vi "Algorithm.vi"(7 "Name(\"\" to use uuid)":string="CSM-Module") -> ()   [LabVIEW 2017, in "Algorithm.lvlib"]
uses:
  Algorithm.lvlib
  b0911fd4-62c2-45de-bc24-cb3c3c9cfef9.vi
  650347b4-7247-415a-b210-2ec4f3372018.vi
  d54ebfec-1730-4eff-a376-8c753df15871.vi
  08833c2f-3e6e-47d2-ae0f-0995abdd27de.vi
  d6c98f61-f9a9-4815-af94-1514c1bd458f.vi
  11c34204-1abb-4db0-9e93-68fba18ec886.vi
  fe892ae6-a90b-4c60-af4d-0c04454fd8c0.vi
  6b00cd4a-b76d-4b12-b38d-c43ef07dbd87.vi
  <userlib>/_NEVSTOP/Communicable State Machine(CSM)/AdvanceAPI/CSM - Revert Arguments-Safe String.vi
  <userlib>/_NEVSTOP/Communicable State Machine(CSM)/_Shared/Trim Single-line Text.vi
  <userlib>/_NEVSTOP/Communicable State Machine(CSM)/AdvanceAPI/CSM - Make String Arguments Safe.vi
  <userlib>/_NEVSTOP/Communicable State Machine(CSM)/AdvanceAPI/CSM - Break Down Multiple States String.vi
  <userlib>/_NEVSTOP/Communicable State Machine(CSM)/AdvanceAPI/CSM - Compact Multiple States.vi
  <userlib>/_NEVSTOP/Communicable State Machine(CSM)/AdvanceAPI/CSM - Keywords.vi
  <userlib>/_NEVSTOP/Communicable State Machine(CSM)/addons/API-String-Arugments-Support/_Support/Query Data as API String Arguments(variant).vi
  <userlib>/_NEVSTOP/Communicable State Machine(CSM)/addons/API-String-Arugments-Support/_Support/Convert API String Arguments to Data(variant).vi
  <userlib>/_NEVSTOP/Communicable State Machine(CSM)/addons/MassData-Parameter/_support/FGV-MassData(lvlibp).vi
  <vilib>/express/express analysis/Spectral/Block/exnSpectralBlock spectral measurements peak poly.vi
  <vilib>/express/express analysis/Spectral/Block/exnSpectralBlock spectral measurements peak array WFM.vi
  <vilib>/express/express analysis/Spectral/Block/exnSpectralBlock spectral measurements RMS poly.vi
  <vilib>/express/express analysis/Spectral/Block/exnSpectralBlock spectral measurements RMS array WFM.vi
  <vilib>/express/express analysis/Spectral/Block/exnSpectralBlock spectral measurements power poly.vi
  <vilib>/express/express analysis/Spectral/Block/exnSpectralBlock spectral measurements power array WFM.vi
  <vilib>/express/express analysis/Spectral/XNode/ExpressSpectralMeasurementsBlockNode.xnode
  <userlib>/_NEVSTOP/Communicable State Machine(CSM)/Communicable State Machine.lvlib
panel:
  out "Source":waveform(dbl)[](graph)
  out "Error Occurred":errorcluster
  out "State History":string
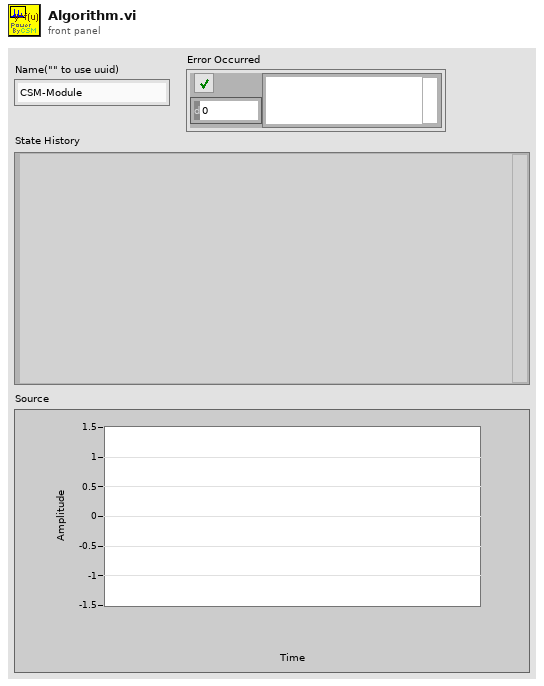
[diagram p1: front panel]
types:
  T1 = enum32{"Invalid", "Standard", "Closed", "Hidden", "Minimized", "Maximized"}
  T2 = enum32{"invalid app kind", "Development System", "Run Time System", "Student Edition", "Embedded LabVIEW", "Evaluation", "Custom"}
  T3 = cluster{"averaging mode":u16, "weighting mode":u16, "number of averages":u32}
  T4 = cluster{"dB On (F)":bool, "unwrap phase (F)":bool, "convert to degree (F)":bool}
  T5 = typedef "Communicable State Machine.lvlib/_CSM_Response Source Message.ctl" = cluster{"‘State":string, "’Arguments":string, "’Error":errorcluster}
  T6 = cluster{"Current VI Reference":refnum<vi>, "Close Panel on Exit?":bool}
  T7 = cluster{"Core":cluster{"Current VI Reference":refnum<vi>, "Close Panel on Exit?":bool}, "Your Boolean data":bool, "Your string data":string}
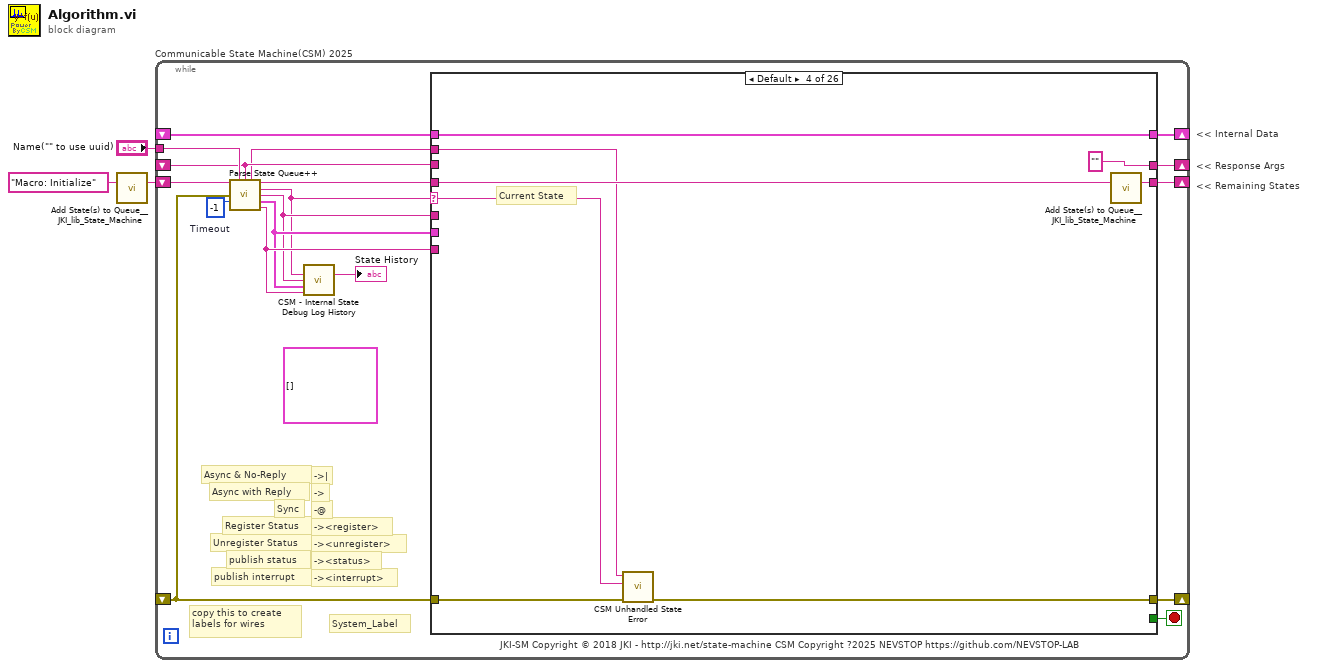
[diagram p0: block diagram]
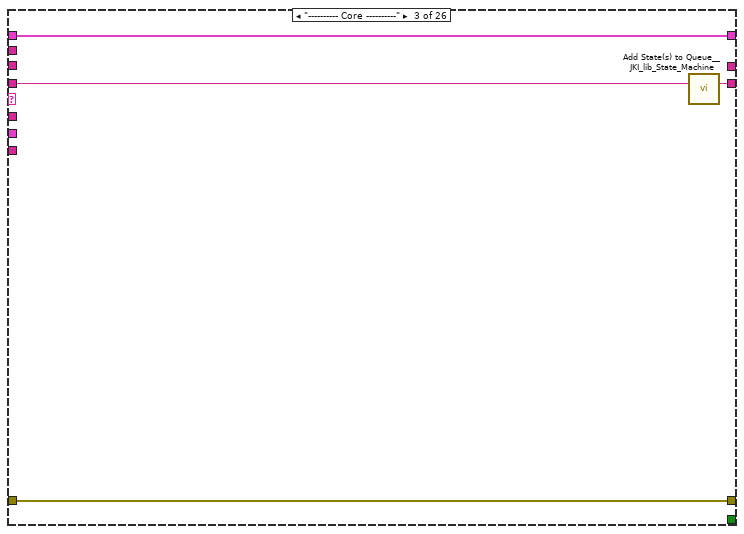
[diagram p4: hidden frame]
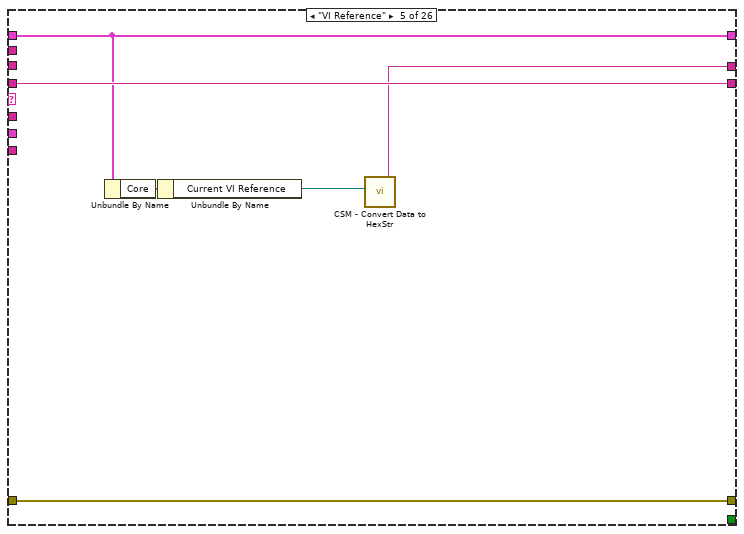
[diagram p5: hidden frame]
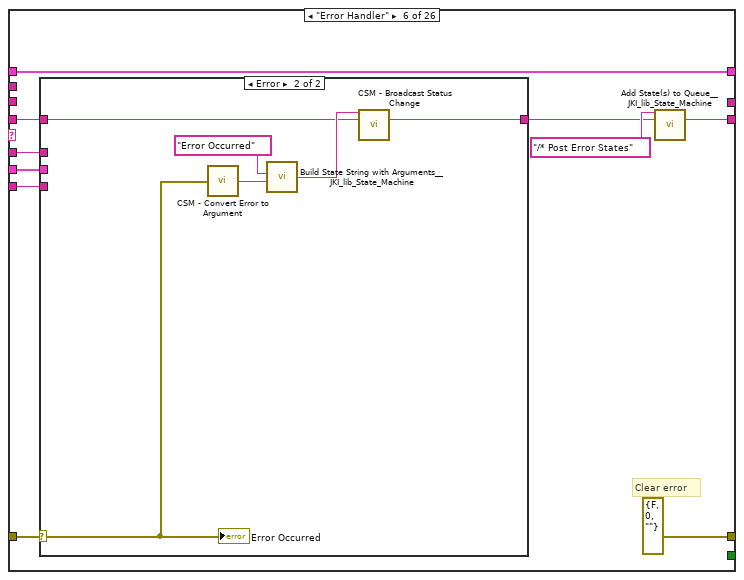
[diagram p6: hidden frame]
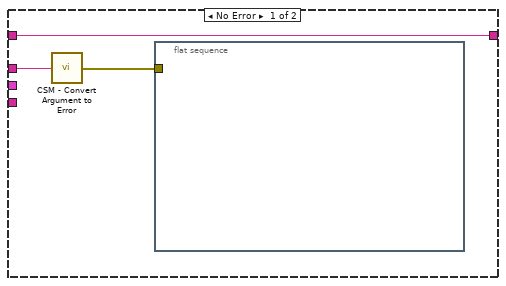
[diagram p7: hidden frame]
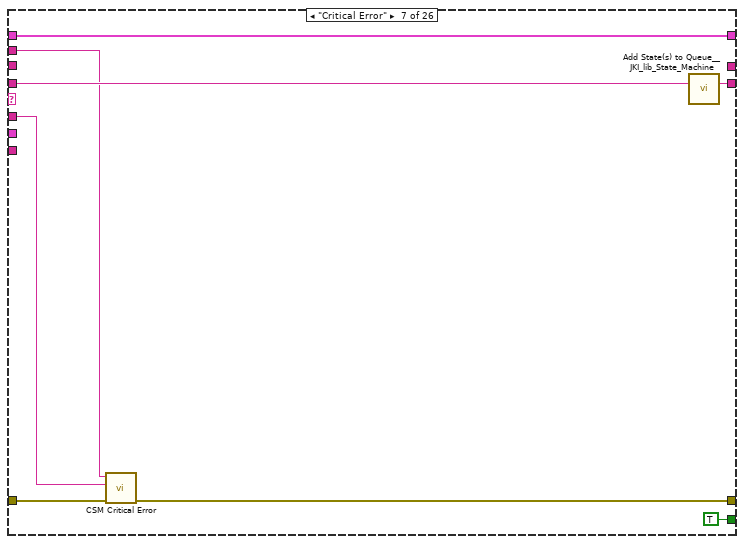
[diagram p8: hidden frame]
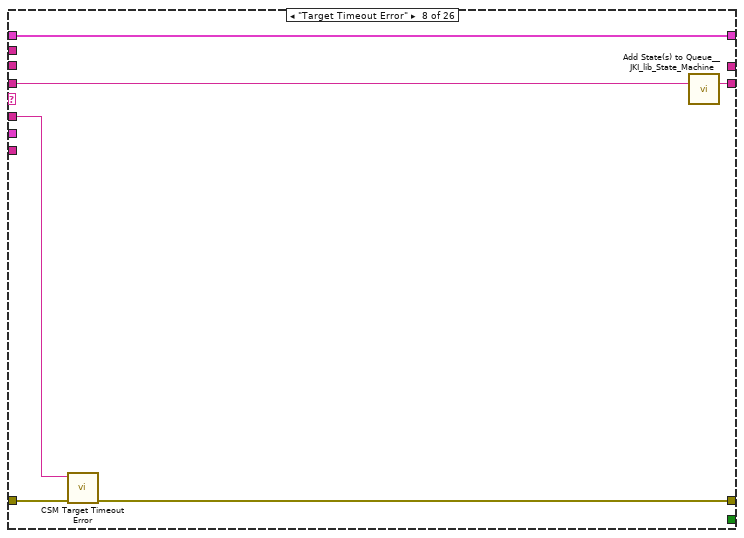
[diagram p9: hidden frame]
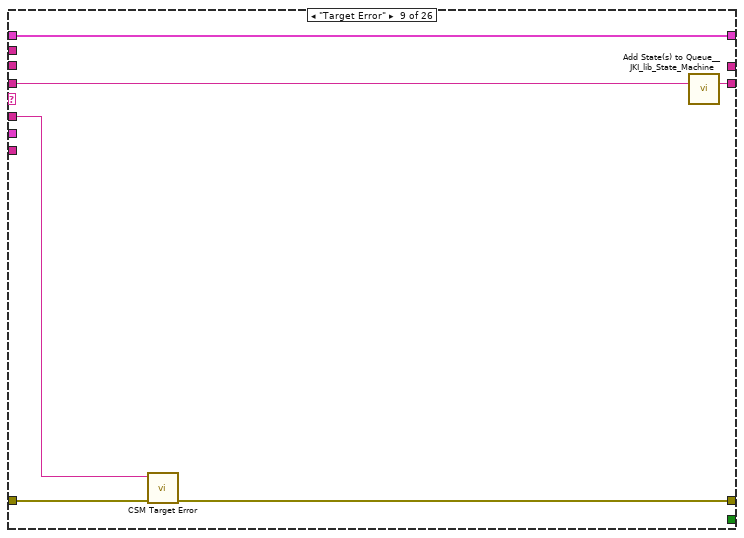
[diagram p10: hidden frame]
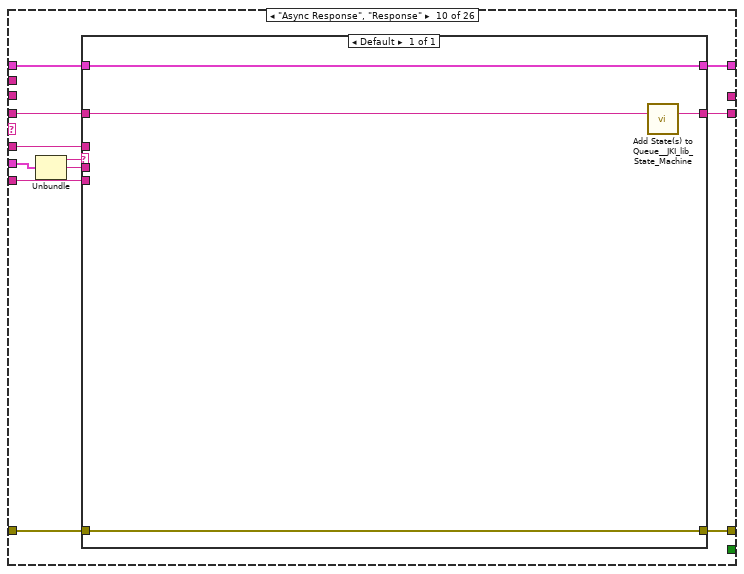
[diagram p11: hidden frame]
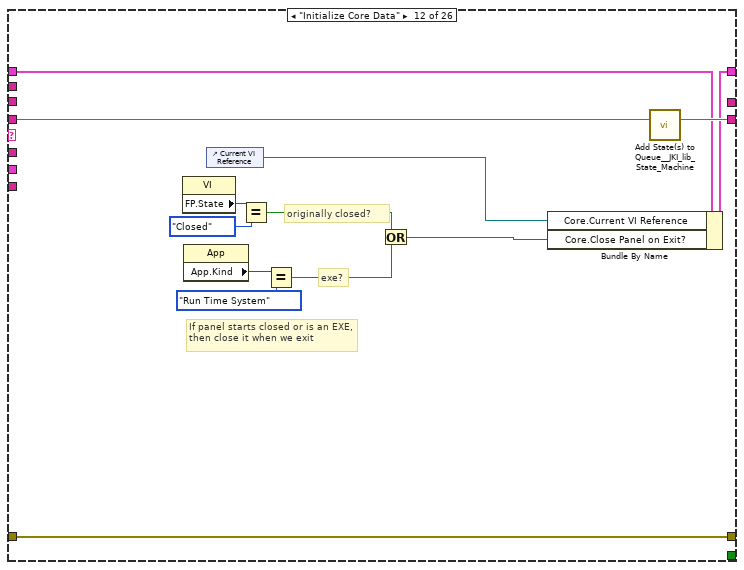
[diagram p13: hidden frame]
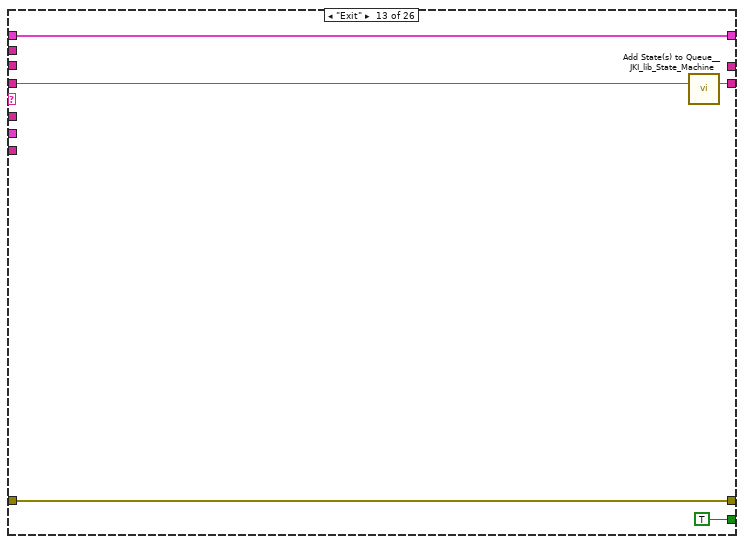
[diagram p14: hidden frame]
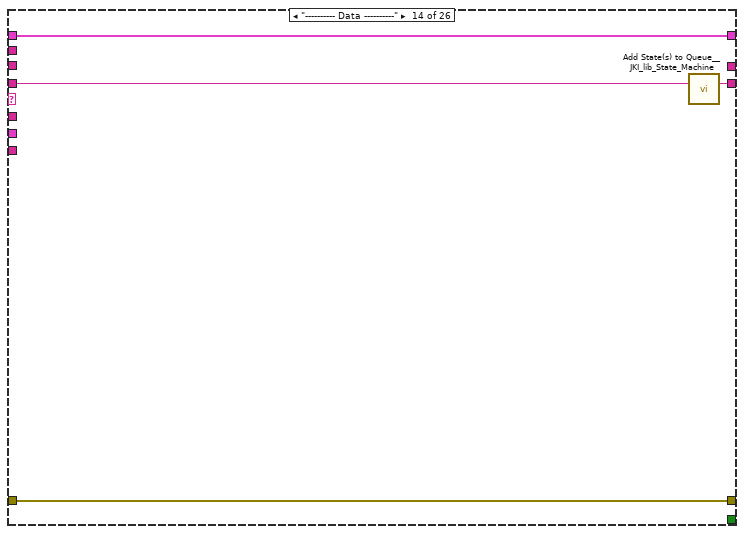
[diagram p15: hidden frame]
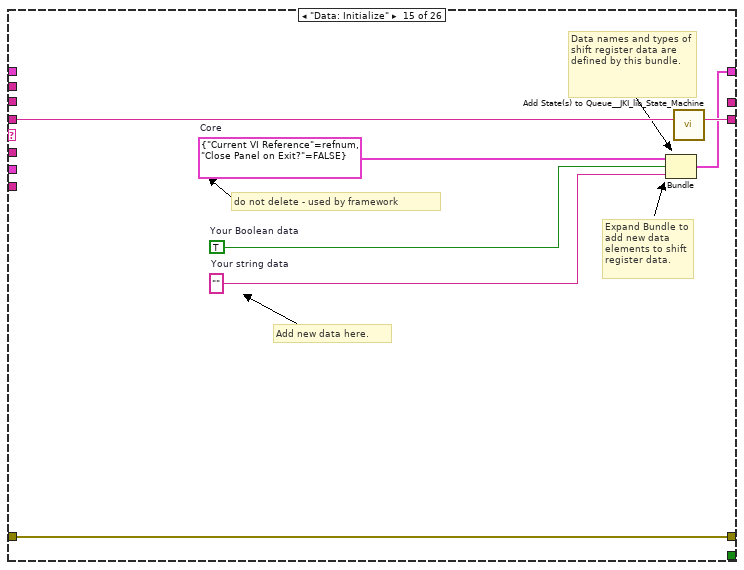
[diagram p16: hidden frame]
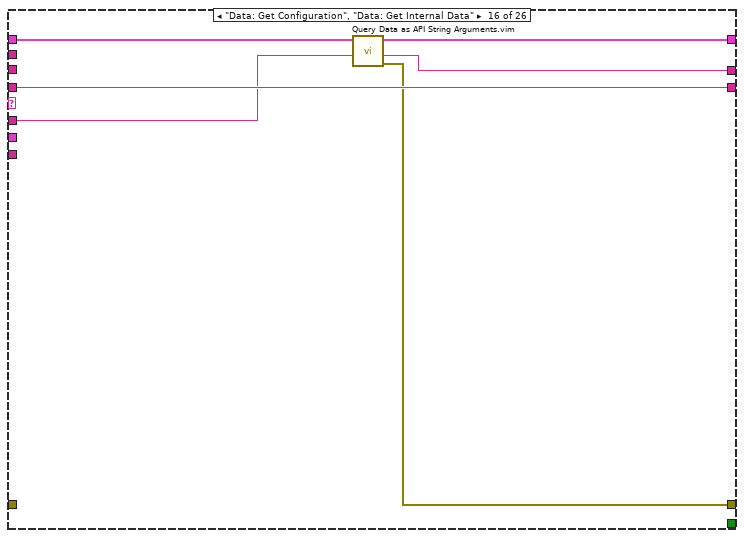
[diagram p17: hidden frame]
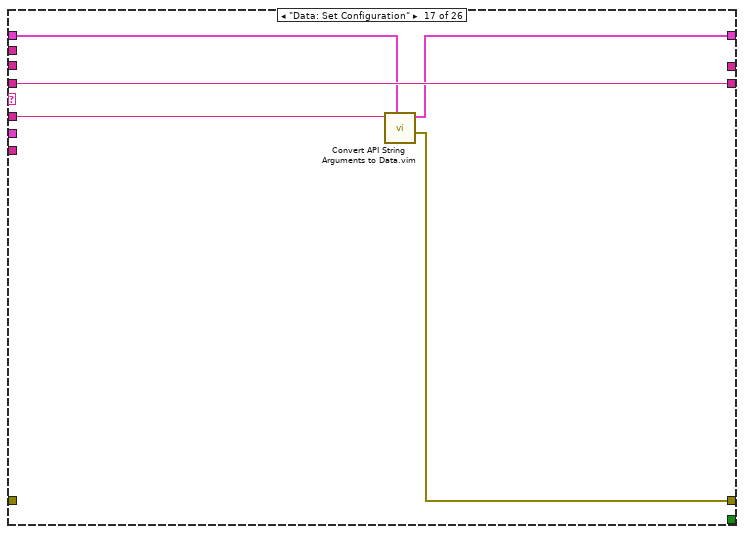
[diagram p18: hidden frame]
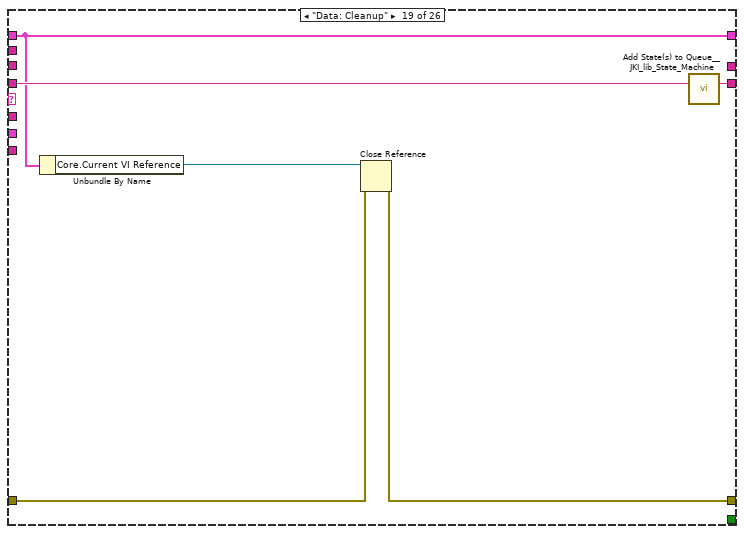
[diagram p20: hidden frame]
diagram:
  # "<< Internal Data"
  # "<< Response Args"
  # "<< Remaining States"
  n1 = call <vilib>:"Add State(s) to Queue__JKI_lib_State_Machine.vi"("State(s) in (\"\")"="Macro: Initialize") -> ("States Out"=w3:string)  [unwired: 14 in]
  n2 = while "Communicable State Machine(CSM) 2025" {
    shift-right: [w16] -> _
    shift-left: _ -> [w15]
    shift-right: [w19] -> _
    shift-left: _ -> [w5]
    shift-right: [w18] -> _
    shift-left: w3 -> [w20]
    tunnel: "Name(\"\" to use uuid)" -> [w12]
    shift-right: [w13] -> _
    shift-left: _ -> [w7]
    stop <- w17 stop-if-true
    (unwired) cluster{"f0":dbl, "df":dbl, "magnitude":dbl[]}[] [] ("FFT - (RMS)")
    w14 = -1  # Timeout
    # "copy this to create labels for wires"
    # "System_Label"
    # "-><interrupt>"
    # "-><status>"
    # "-><unregister>"
    # "-><register>"
    # "-@"
    # "->"
    # "->|"
    # "publish interrupt"
    # "publish status"
    # "Unregister Status"
    # "Register Status"
    # "Sync"
    # "Async with Reply"
    # "Async & No-Reply"
    # "JKI-SM Copyright © 2018 JKI - http://jki.net/state-machine CSM Copyright ?2025 NEVSTOP https://github.com/NEVSTOP-LAB"
    n3 = call <userlib>:"Parse State Queue++.vi"("State Queue"=w20, "Name (\"\" to Use UUID)"=w12, "Response Arguments"=w7, "Previous Error"=w5, "Dequeue (1 ms)"=w14) -> ("Name Used"=w6:string, "Remaining States"=w21:string, "Current State"=w8:string, "Arguments"=w9:string, "Additional Information"=w10:T5, "Source CSM"=w11:string)  [unwired: 5 in]
    n4 = call <userlib>:"CSM - Internal State Debug Log History.vi"("State"=w8, "Arguments (\"\")"=w9, ">> Response Source Message >>"=w10, "Source (\"\")"=w11) -> ("Debug Log"=→"State History":string)  [unwired: 11 in]
    n5 = case shown="Default" w8 {
      selector: w8 -> [_ _ _ w34 _ _ _ _ _ _ _ _ _ _ _ _ _ _ _ _ _ _ _ _ _ _]
      tunnel: w21 -> [w22 w26 w31 w38 w44 w49 w71 w77 w83 w88 w101 w115 w120 w124 w131 w137 w142 w144 w151 w155 w160 w165 w167 w178 w198 w218]
      tunnel: w9 -> [_ _ _ _ _ w48 w66 w74 w80 w87 _ _ _ _ _ w132 w141 _ _ _ _ _ _ w175 w195 w215]
      tunnel: w15 -> [w23 w25 w28 w36 w43 w54 w69 w75 w81 w89 w100 w108 w118 w121 _ w136 w140 w143 w146 w152 w157 w162 w166 w177 w197 w217]
      tunnel: [w24 w27 w29 w32 w45 errorcluster {"status"=FALSE, "code"=0, "source"=""} ("error out") w65 w73 w79 w92 w102 w112 w117 w122 w128 w133 w138 w145 w147 w153 w158 w163 w168 w171 w191 w211] -> w19
      tunnel: w5 -> [w24 w27 w29 w39 w45 w52 w72 w78 w84 w93 w102 w112 w117 w122 w128 _ _ w145 w148 w153 w158 w163 w168 _ _ _]
      tunnel: [w22 w26 w30 w37 w44 w50 w70 w76 w82 w90 w101 w114 w119 w123 w130 w137 w142 w144 w150 w154 w159 w164 w167 w178 w198 w218] -> w18
      tunnel: [_ _ _ _ _ _ TRUE _ _ _ _ _ TRUE _ _ _ _ _ _ _ _ _ _ _ _ _] -> w17
      tunnel: [w23 w25 w28 w36 w43 w54 w69 w75 w81 w91 w100 w113 w118 w121 w129 w135 w139 w143 w146 w152 w157 w162 w166 w177 w197 w217] -> w16
      tunnel: w11 -> [_ _ _ _ _ w47 _ _ _ w85 _ _ _ _ _ _ _ _ _ _ _ _ _ _ _ _]
      tunnel: w10 -> [_ _ _ _ _ w46 _ _ _ w86 _ _ _ _ _ _ _ _ _ _ _ _ _ _ _ _]
      tunnel: [_ _ _ "" w40 _ _ _ _ _ _ _ _ _ _ w134 _ _ _ _ _ _ _ w170 w190 w210] -> w13
      tunnel: w6 -> [_ _ _ w33 _ _ w67 _ _ _ _ _ _ _ _ _ _ _ _ _ _ _ _ _ _ _]
      tunnel: w7 -> [_ _ _ _ _ _ _ _ _ _ _ _ _ _ _ _ _ _ _ _ _ _ _ _ _ _]
      frame "", "Idle" {
      }
      frame "CSM Documentation" {
        # "CSM Documentation"
      }
      frame "---------- Core ----------" {
        n6 = call <vilib>:"Add State(s) to Queue__JKI_lib_State_Machine.vi"("State(s) in (\"\")"=w31) -> ("States Out"=w30:string)  [unwired: 14 in]
      }
      frame Default {
        # "Current State"
        n7 = call <userlib>:"CSM Unhandled State Error.vi"("error in (no error)"=w39, "Undefined State"=w34, "CSM Name"=w33) -> ("error out"=w32:errorcluster)  [unwired: 8 in]
        n8 = call <vilib>:"Add State(s) to Queue__JKI_lib_State_Machine.vi"("State(s) in (\"\")"=w38) -> ("States Out"=w37:string)  [unwired: 14 in]
      }
      frame "VI Reference" {
        n9 = Unbundle By Name(w43) -> ("Core"=w42:T6)
        n10 = Unbundle By Name(w42) -> ("Current VI Reference"=w41:refnum<vi>)
        n11 = call <userlib>:"CSM - Convert Data to HexStr.vi"("Variant"=w41) -> ("HEX String (0-9,A-F)"=w40:string)  [unwired: 8 in]
      }
      frame "Error Handler" {
        # "Clear error"
        n12 = case shown="Error" w52 {
          selector: w52 -> [_ w59]
          tunnel: [w58 w61] -> w51
          tunnel: w49 -> [w58 w60]
          tunnel: w48 -> [w57 _]
          tunnel: w47 -> [_ _]
          tunnel: w46 -> [_ _]
          frame No Error {
            n13 = call <userlib>:"CSM - Convert Argument to Error.vi"("Argument"=w57) -> ("Error"=w56:errorcluster)  [unwired: 4 in]
            n14 = flat-sequence {
              tunnel: w56 -> [_]
              frame #0 {
              }
            }
          }
          frame Error {
            n15 = call <userlib>:"CSM - Convert Error to Argument.vi"("Error"=w59) -> ("Argument"=w63:string)  [unwired: 4 in]
            n16 = call <vilib>:"Build State String with Arguments__JKI_lib_State_Machine.vi"("Arguments (\"\")"=w63, "State"="Error Occurred" ("Status with Arguments")) -> ("State with Arguments"=w62:string)  [unwired: 4 in]
            n17 = call <userlib>:"CSM - Broadcast Status Change.vi"("Status With Arguments"=w62, "State Queue"=w60) -> ("Remaining States"=w61:string)  [unwired: 13 in]
            "Error Occurred" <- w59
          }
        }
        n18 = call <vilib>:"Add State(s) to Queue__JKI_lib_State_Machine.vi"("State(s) in Front (\"\")"="/* Post Error States", "State(s) in (\"\")"=w51) -> ("States Out"=w50:string)  [unwired: 13 in]
      }
      frame "Critical Error" {
        n19 = call <userlib>:"CSM Critical Error.vi"("error in (no error)"=w72, "Arugments (As Reason)"=w66, "CSM Name"=w67) -> ("error out"=w65:errorcluster)  [unwired: 8 in]
        n20 = call <vilib>:"Add State(s) to Queue__JKI_lib_State_Machine.vi"("State(s) in (\"\")"=w71) -> ("States Out"=w70:string)  [unwired: 14 in]
      }
      frame "Target Timeout Error" {
        n21 = call <userlib>:"CSM Target Timeout Error.vi"("error in (no error)"=w78, "Arguments (As CSM Name)"=w74) -> ("error out"=w73:errorcluster)  [unwired: 9 in]
        n22 = call <vilib>:"Add State(s) to Queue__JKI_lib_State_Machine.vi"("State(s) in (\"\")"=w77) -> ("States Out"=w76:string)  [unwired: 14 in]
      }
      frame "Target Error" {
        n23 = call <userlib>:"CSM Target Error.vi"("error in (no error)"=w84, "Arguments (As CSM Name)"=w80) -> ("error out"=w79:errorcluster)  [unwired: 9 in]
        n24 = call <vilib>:"Add State(s) to Queue__JKI_lib_State_Machine.vi"("State(s) in (\"\")"=w83) -> ("States Out"=w82:string)  [unwired: 14 in]
      }
      frame "Async Response", "Response" {
        n25 = Unbundle(w86) -> ("‘State"=w95:string, "’Arguments"=w94:string)  [unwired: 1 out]
        n26 = case shown="Default" w95 {
          tunnel: [w96] -> w90
          tunnel: w88 -> [w97]
          tunnel: [w99] -> w91
          tunnel: w89 -> [w99]
          tunnel: [w98] -> w92
          tunnel: w93 -> [w98]
          tunnel: w85 -> [_]
          tunnel: w87 -> [_]
          tunnel: w94 -> [_]
          frame Default {
            n27 = call <vilib>:"Add State(s) to Queue__JKI_lib_State_Machine.vi"("State(s) in (\"\")"=w97) -> ("States Out"=w96:string)  [unwired: 14 in]
          }
        }
      }
      frame "Async Message Posted" {
      }
      frame "Initialize Core Data" {
        # "originally closed?"
        # "exe?"
        # "If panel starts closed or is an EXE, then close it when we exit"
        n28 = property class="VI"() -> ("FP.State"=w105:T1)  [unwired: 2 in, 2 out]
        n29 = property class="App"() -> ("App.Kind"=w111:T2)  [unwired: 2 in, 2 out]
        n30 = control-ref of="Current VI Reference"() -> (w106:refnum<vi>)
        n31 = Equal?(x=w105, y=T1."Closed" ("Front Panel Window:State")) -> (x = y?=w103:bool)
        n32 = Equal?(x=w111, y=T2."Run Time System" ("Application:Kind")) -> (x = y?=w109:bool)
        n33 = Or(x=w103, y=w109) -> (x .or. y?=w107:bool)
        n34 = Bundle By Name(cluster=w108, "Core.Current VI Reference"=w106, "Core.Close Panel on Exit?"=w107) -> (w113:T7)
        n35 = call <vilib>:"Add State(s) to Queue__JKI_lib_State_Machine.vi"("State(s) in (\"\")"=w115) -> ("States Out"=w114:string)  [unwired: 14 in]
      }
      frame "Exit" {
        n36 = call <vilib>:"Add State(s) to Queue__JKI_lib_State_Machine.vi"("State(s) in (\"\")"=w120) -> ("States Out"=w119:string)  [unwired: 14 in]
      }
      frame "---------- Data ----------" {
        n37 = call <vilib>:"Add State(s) to Queue__JKI_lib_State_Machine.vi"("State(s) in (\"\")"=w124) -> ("States Out"=w123:string)  [unwired: 14 in]
      }
      frame "Data: Initialize" {
        w125 = T6 {"Current VI Reference"=refnum, "Close Panel on Exit?"=FALSE}  # Core
        w127 = TRUE  # Your Boolean data
        w126 = ""  # Your string data
        # "do not delete - used by framework"
        # "Expand Bundle to add new data elements to shift register data."
        # "Add new data here."
        # "Data names and types of shift register data are defined by this bundle."
        n38 = Bundle("Core"=w125, "Your Boolean data"=w127, "Your string data"=w126) -> (w129:T7)  [unwired: 1 in]
        n39 = call <vilib>:"Add State(s) to Queue__JKI_lib_State_Machine.vi"("State(s) in (\"\")"=w131) -> ("States Out"=w130:string)  [unwired: 14 in]
      }
      frame "Data: Get Configuration", "Data: Get Internal Data" {
        n40 = call "Query Data as API String Arguments.vim"("Name"=w132, "Cluster Data"=w136) -> ("error"=w133:errorcluster, "API String"=w134:string, "Cluster Data (dup)"=w135:T7)  [unwired: 7 in]
      }
      frame "Data: Set Configuration" {
        n41 = call "Convert API String Arguments to Data.vim"("Reference Type"=w140, "API String"=w141) -> ("error out"=w138:errorcluster, "Data"=w139:T7)  [unwired: 6 in]
      }
      frame "Data: Update Indicators" {
      }
      frame "Data: Cleanup" {
        n42 = Unbundle By Name(w146) -> ("Core.Current VI Reference"=w149:refnum<vi>)
        n43 = Close Reference(reference=w149, error in (no error)=w148) -> (error out=w147:errorcluster)
        n44 = call <vilib>:"Add State(s) to Queue__JKI_lib_State_Machine.vi"("State(s) in (\"\")"=w151) -> ("States Out"=w150:string)  [unwired: 14 in]
      }
      frame "---------- Macro ----------" {
        n45 = call <vilib>:"Add State(s) to Queue__JKI_lib_State_Machine.vi"("State(s) in (\"\")"=w155) -> ("States Out"=w154:string)  [unwired: 14 in]
      }
      frame "Macro: Initialize" {
        n46 = call <vilib>:"Add State(s) to Queue__JKI_lib_State_Machine.vi"("State(s) in Front (\"\")"="Data: Initialize\nInitialize Core Data\nData: Update Indicators", "State(s) in (\"\")"=w160) -> ("States Out"=w159:string)  [unwired: 13 in]
      }
      frame "Macro: Exit" {
        n47 = call <vilib>:"Add State(s) to Queue__JKI_lib_State_Machine.vi"("State(s) in Front (\"\")"="Data: Cleanup\nExit", "State(s) in (\"\")"=w165) -> ("States Out"=w164:string)  [unwired: 13 in]
      }
      frame "---------- API ----------" {
      }
      frame "API: FFT(Peak)" {
        n48 = call "CSM - Convert Argument to MassData.vim"("Type"=waveform(dbl)[] [] ("data"), "MassData Argument"=w175) -> ("error out"=w174:errorcluster, "Data"=w169:waveform(dbl)[])  [unwired: 6 in]
        n49 = xnode "Spectral Measurements"("Signals"=w169, "error in (no error)"=w174) -> ("FFT - (Peak)"=w173:cluster{"f0":dbl, "df":dbl, "magnitude":dbl[]}[], "error out"=w172:errorcluster)  [unwired: 1 out]
        n50 = local write "Source"(w169) -> ()
        n51 = call "CSM - Convert MassData to Argument.vim"("error in (no error)"=w172, "Data"=w173) -> ("error out"=w171:errorcluster, "MassData Argument"=w170:string)  [unwired: 6 in]
      }
      frame "API: FFT(RMS)" {
        n52 = call "CSM - Convert Argument to MassData.vim"("Type"=waveform(dbl)[] [] ("data"), "MassData Argument"=w195) -> ("error out"=w194:errorcluster, "Data"=w189:waveform(dbl)[])  [unwired: 6 in]
        n53 = xnode "Spectral Measurements"("Signals"=w189, "error in (no error)"=w194) -> ("FFT - (RMS)"=w193:cluster{"f0":dbl, "df":dbl, "magnitude":dbl[]}[], "error out"=w192:errorcluster)  [unwired: 1 out]
        n54 = local write "Source"(w189) -> ()
        n55 = call "CSM - Convert MassData to Argument.vim"("error in (no error)"=w192, "Data"=w193) -> ("error out"=w191:errorcluster, "MassData Argument"=w190:string)  [unwired: 6 in]
      }
      frame "API: Power Spectrum" {
        n56 = call "CSM - Convert Argument to MassData.vim"("Type"=waveform(dbl)[] [] ("data"), "MassData Argument"=w215) -> ("error out"=w214:errorcluster, "Data"=w209:waveform(dbl)[])  [unwired: 6 in]
        "Source" <- w209
        n57 = xnode "Spectral Measurements"("Signals"=w209, "error in (no error)"=w214) -> ("Power Spectrum"=w213:cluster{"f0":dbl, "df":dbl, "magnitude":dbl[]}[], "error out"=w212:errorcluster)
        n58 = call "CSM - Convert MassData to Argument.vim"("error in (no error)"=w212, "Data"=w213) -> ("error out"=w211:errorcluster, "MassData Argument"=w210:string)  [unwired: 6 in]
      }
    }
  }
